vi "Save As Sif.vi"(11 "path":string) -> (2 "function return":u32, 3 "path out":string)   [LabVIEW 2018, in "Copy of Andor SDK.lvlib"]
doc: "EXPNETTYPE unsigned int WINAPI SaveAsSif(char * path);"
uses:
  Copy of Andor SDK.lvlib
  <userlib>/Andor SDK/ATMCD32D.dll
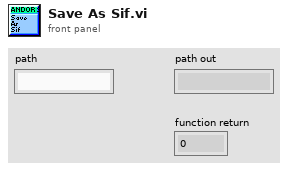
[diagram p1: front panel]
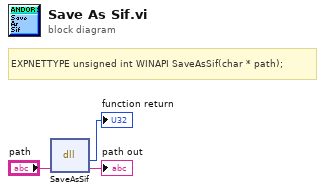
[diagram p0: block diagram]
diagram:
  # "EXPNETTYPE unsigned int WINAPI SaveAsSif(char * path);"
  n1 = dll-call lib="C:/Program Files (x86)/National Instruments/LabVIEW 2018/user.lib/Andor SDK/ATMCD32D.*" fn="SaveAsSif"("path"="path") -> (→"function return":u32, "path"=→"path out":string)  [unwired: 3 in, 2 out]
